vi "Save File Look for File Number.vi"(8 "Error In":errorcluster, 11 "Old path":path) -> (0 "Error Out":errorcluster, 1 "Last Portion of File Name":string, 2 "File Name (Before \"FILE\")":string, 3 "Base Path (No File Name)":path)   [LabVIEW 2016, in "Save File.lvlib"]
uses:
  Save File.lvlib
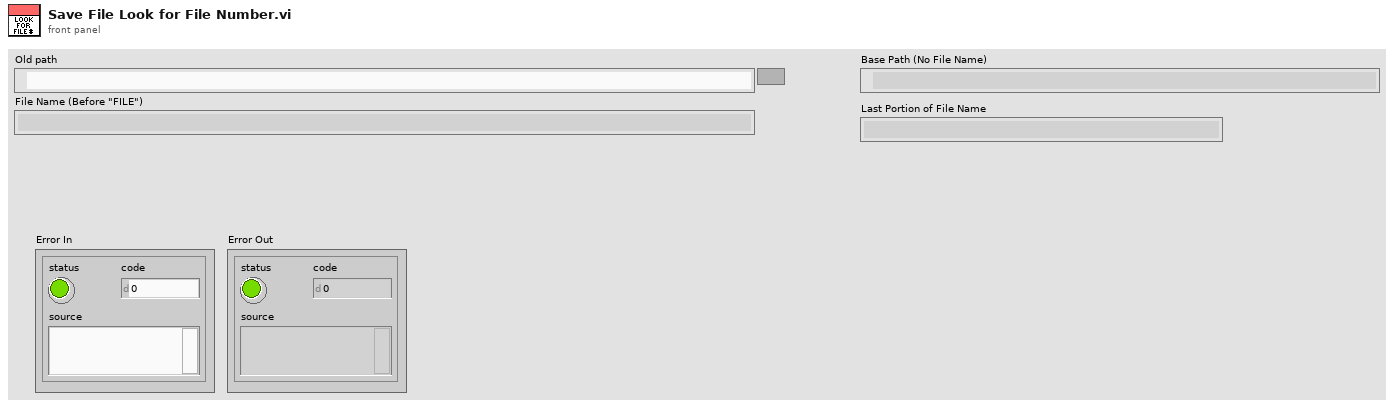
[diagram p1: front panel]
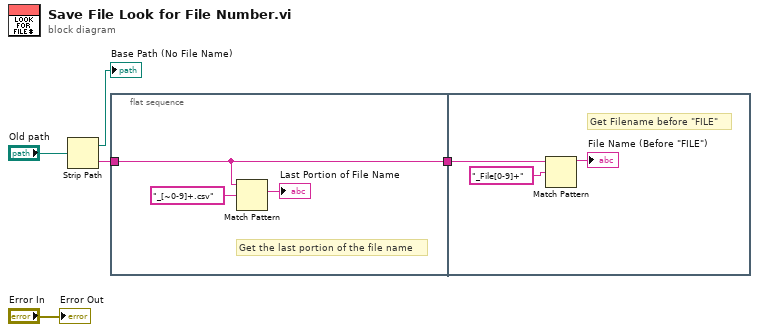
[diagram p0: block diagram]
diagram:
  n1 = Strip Path(path="Old path") -> (stripped path=→"Base Path (No File Name)":path, name=w3:string)
  n2 = flat-sequence {
    tunnel: w3 -> [w6]
    tunnel: [w6] -> w2
    tunnel: w2 -> [w9]
    frame #0 {
      # "Get the last portion of the file name"
      n3 = Match Pattern(string=w6, regular expression="_[~0-9]+.csv") -> (match substring=→"Last Portion of File Name":string)  [unwired: 1 in, 3 out]
    }
    frame #1 {
      # "Get Filename before \"FILE\""
      n4 = Match Pattern(string=w9, regular expression="_File[0-9]+") -> (before substring=→"File Name (Before \"FILE\")":string)  [unwired: 1 in, 3 out]
    }
  }
  "Error Out" <- "Error In"
